vi "lock-in input sweep_1022D.vi"() -> ()   [LabVIEW 2022 SP3]
uses:
  <vilib>/Analysis/baseanly.llb/Mean (DBL).vi
  <vilib>/Utility/file.llb/Write Delimited Spreadsheet (DBL).vi
  <vilib>/Analysis/NI_AALBase.lvlib
panel:
  in  "Series Resistance":string="20kOhm"
  in  "Temperature \n& Field Function":bool=TRUE
  in  "Field Approach":i32(ring) items=["Linear", "NoOvershoot", "Oscillate"]
  in  "F Rate (Oe/s)":dbl=100.0 format="%#_13g"
  in  "Set F (Oe)":dbl format="%#_13g"
  in  "Mode":i32(ring) items=["Persistent", "Driven"]
  in  "Temperature Approach":i32(ring)=1 items=["FastSettle", "NoOvershoot"]
  in  "T  Rate (K/min)":dbl=10.0
  in  "Set  T  (K)":dbl=2.0
  in  "WaitForField":bool=TRUE
  in  "WaitForTemperature":bool=TRUE
  out "Temperature Status":i32(ring) items=["TemperatureUnknown"=0, "Stable"=1, "Tracking"=2, "Near"=5, "Chasing"=6, "Filling"=7, "Standby"=10, "Disabled"=13, "ImpedanceNotFunction"=14, "TempFailure"=15]
  out "Field Status":i32(ring) items=["MagnetUnknown"=0, "StablePersistent"=1, "WarmingSwitch"=2, "CoolingSwitch"=3, "StableDriven"=4, "Iterating"=5, "Charging"=6, "Discharging"=7, "CurrentError"=8, "MagnetFailure"=15]
  out "Field":dbl
  in  "Delay":dbl=5.0
  out "Temperature":dbl
  in  "Remote":bool=TRUE
  in  "IP Address":string="169.254.170.239"
  out "Measuring":bool
  in  "A Low Pass Filter Slope":u8(ring)=2 items=["6 dB/oct", "12 dB/oct", "18 db/oct", "24 dB/oct"]
  in  "B Low Pass Filter Slope":u8(ring)=2 items=["6 dB/oct", "12 dB/oct", "18 db/oct", "24 dB/oct"]
  in  "B Reference Source":u8(ring) items=["External", "Internal", "Internal Sweep", "Channel-A"]
  in  "B Time Constant":u8(ring)=9 items=["10 us", "30 us", "100 us", "300 us", "1 ms", "3 ms", "10 ms", "30 ms", "100 ms", "300 ms", "1 s", "3 s", "10 s", "30 s", "100 s", "300 s", "1 ks", "3 ks"]
  in  "Enable Sync Filter B (open when f<200Hz)":bool
  in  "B Sensitivity":u16(ring)=17 items=["1 nV/fA", "2 nV/fA", "5 nV/fA", "10 nV/fA", "20 nV/fA", "50 nV/fA", "100 nV/fA", "200 nV/fA", "500 nV/fA", "1 uV/pA", "2 uV/pA", "5 uV/pA", "10 uV/pA", "20 uV/pA", "50 uV/pA", "100 uV/pA", "200 uV/pA", "500 uV/pA", "1 mV/nA", "2 mV/nA", "5 mV/nA", "10 mV/nA", "20 mV/nA", "50 mV/nA", "100 mV/nA", "200 mV/nA", "500 mV/nA", "1 V/uA"]
  in  "A Sensitivity":u16(ring)=23 items=["1 nV/fA", "2 nV/fA", "5 nV/fA", "10 nV/fA", "20 nV/fA", "50 nV/fA", "100 nV/fA", "200 nV/fA", "500 nV/fA", "1 uV/pA", "2 uV/pA", "5 uV/pA", "10 uV/pA", "20 uV/pA", "50 uV/pA", "100 uV/pA", "200 uV/pA", "500 uV/pA", "1 mV/nA", "2 mV/nA", "5 mV/nA", "10 mV/nA", "20 mV/nA", "50 mV/nA", "100 mV/nA", "200 mV/nA", "500 mV/nA", "1 V/uA"]
  in  "Enable Sync Filter A (open when f<200Hz)":bool
  in  "A Time Constant":u8(ring)=9 items=["10 us", "30 us", "100 us", "300 us", "1 ms", "3 ms", "10 ms", "30 ms", "100 ms", "300 ms", "1 s", "3 s", "10 s", "30 s", "100 s", "300 s", "1 ks", "3 ks"]
  out "XY Graph 4":cluster{dbl[], dbl[]}(graph)
  in  "Phase B":u16(ring)=9 items=["X", "Y", "R", "Theta", "Frequency", "Noise", "Xh1", "Yh1", "Rh1", "Theta h1", "Xh2", "Yh2", "Rh2", "Theta h2"]
  in  "Parameter B":u16(ring)=8 items=["X", "Y", "R", "Theta", "Frequency", "Noise", "Xh1", "Yh1", "Rh1", "Theta h1", "Xh2", "Yh2", "Rh2", "Theta h2"]
  out "phase B":dbl
  in  "Clear Plot B":bool
  out "XY Graph 3":cluster{dbl[], dbl[]}(graph)
  out "para2 Measurement":dbl=1.49013e-07
  out "XY Graph 2":cluster{dbl[], dbl[]}(graph)
  in  "B Sample time (s)":dbl=0.001 min=0.001 max=100.0 step=0.001
  in  "A Sample time (s)":dbl=0.001 min=0.001 max=100.0 step=0.001
  in  "Phase A":u16(ring)=3 items=["X", "Y", "R", "Theta", "Frequency", "Noise", "Xh1", "Yh1", "Rh1", "Theta h1", "Xh2", "Yh2", "Rh2", "Theta h2"]
  in  "Parameter A":u16(ring)=2 items=["X", "Y", "R", "Theta", "Frequency", "Noise", "Xh1", "Yh1", "Rh1", "Theta h1", "Xh2", "Yh2", "Rh2", "Theta h2"]
  in  "stabilization(S)":dbl=1.0 format="%#_13g"
  in  "B frequency":dbl=267.77 format="%#_13g"
  in  "B Input Connection (0: Single-Ended)":u16(ring)=1 items=["Single-Ended Voltage", "Differential Voltage", "1 MOhm Current Gain", "100 MOhm Current Gain"]
  in  "B harmonic 1":u8=2
  in  "B harmonic 2":u8=3
  in  "B reference Manual Phase  2":dbl=-59.75
  in  "auto phase B":bool=TRUE
  in  "A frequency":dbl=267.77 format="%#_13g"
  in  "A Input Connection (0: Single-Ended)":u16(ring)=1 items=["Single-Ended Voltage", "Differential Voltage", "1 MOhm Current Gain", "100 MOhm Current Gain"]
  in  "A harmonic 1":u8=2
  in  "A harmonic 2":u8=3
  in  "A reference Manual Phase":dbl=-59.75
  in  "auto phase A":bool=TRUE
  in  "A Reference Source":u8(ring)=1 items=["External", "Internal", "Internal Sweep"]
  out "phase A":dbl
  out "loop run":i32
  in  "loop #":i32=1
  in  "Save data or not":bool=TRUE
  in  "path (folder + filename)":string="G:\\My Drive\\Opticool\\Measurement\\NLH\\f dependence\\TaI21_A1615_B166_267Hz"
  in  "Clear Plot A":bool
  out "XY Graph":cluster{dbl[], dbl[]}(graph)
  out "para1 Measurement":dbl=1.49013e-07
  out "Sine voltage":dbl format="%#_13g"
  in  "GATE STEP(mv)":i32=20
  in  "Sine Low Value (default 0V)":dbl=0.1
  in  "Sine High Value (0.001-5V)":dbl=3.5
  in  "lockin waiting (s)":dbl=0.1 format="%#_13g"
  in  "LOCKIN address":refnum<visa-resource-name>="COM3"
  # "Lock-in Setting"
  # "Channel B"
  # "Channel A"
  # "Mesurement"
  # "Sine Sweep Setting (Channel A)"
  # "Temprature and Field Setting"
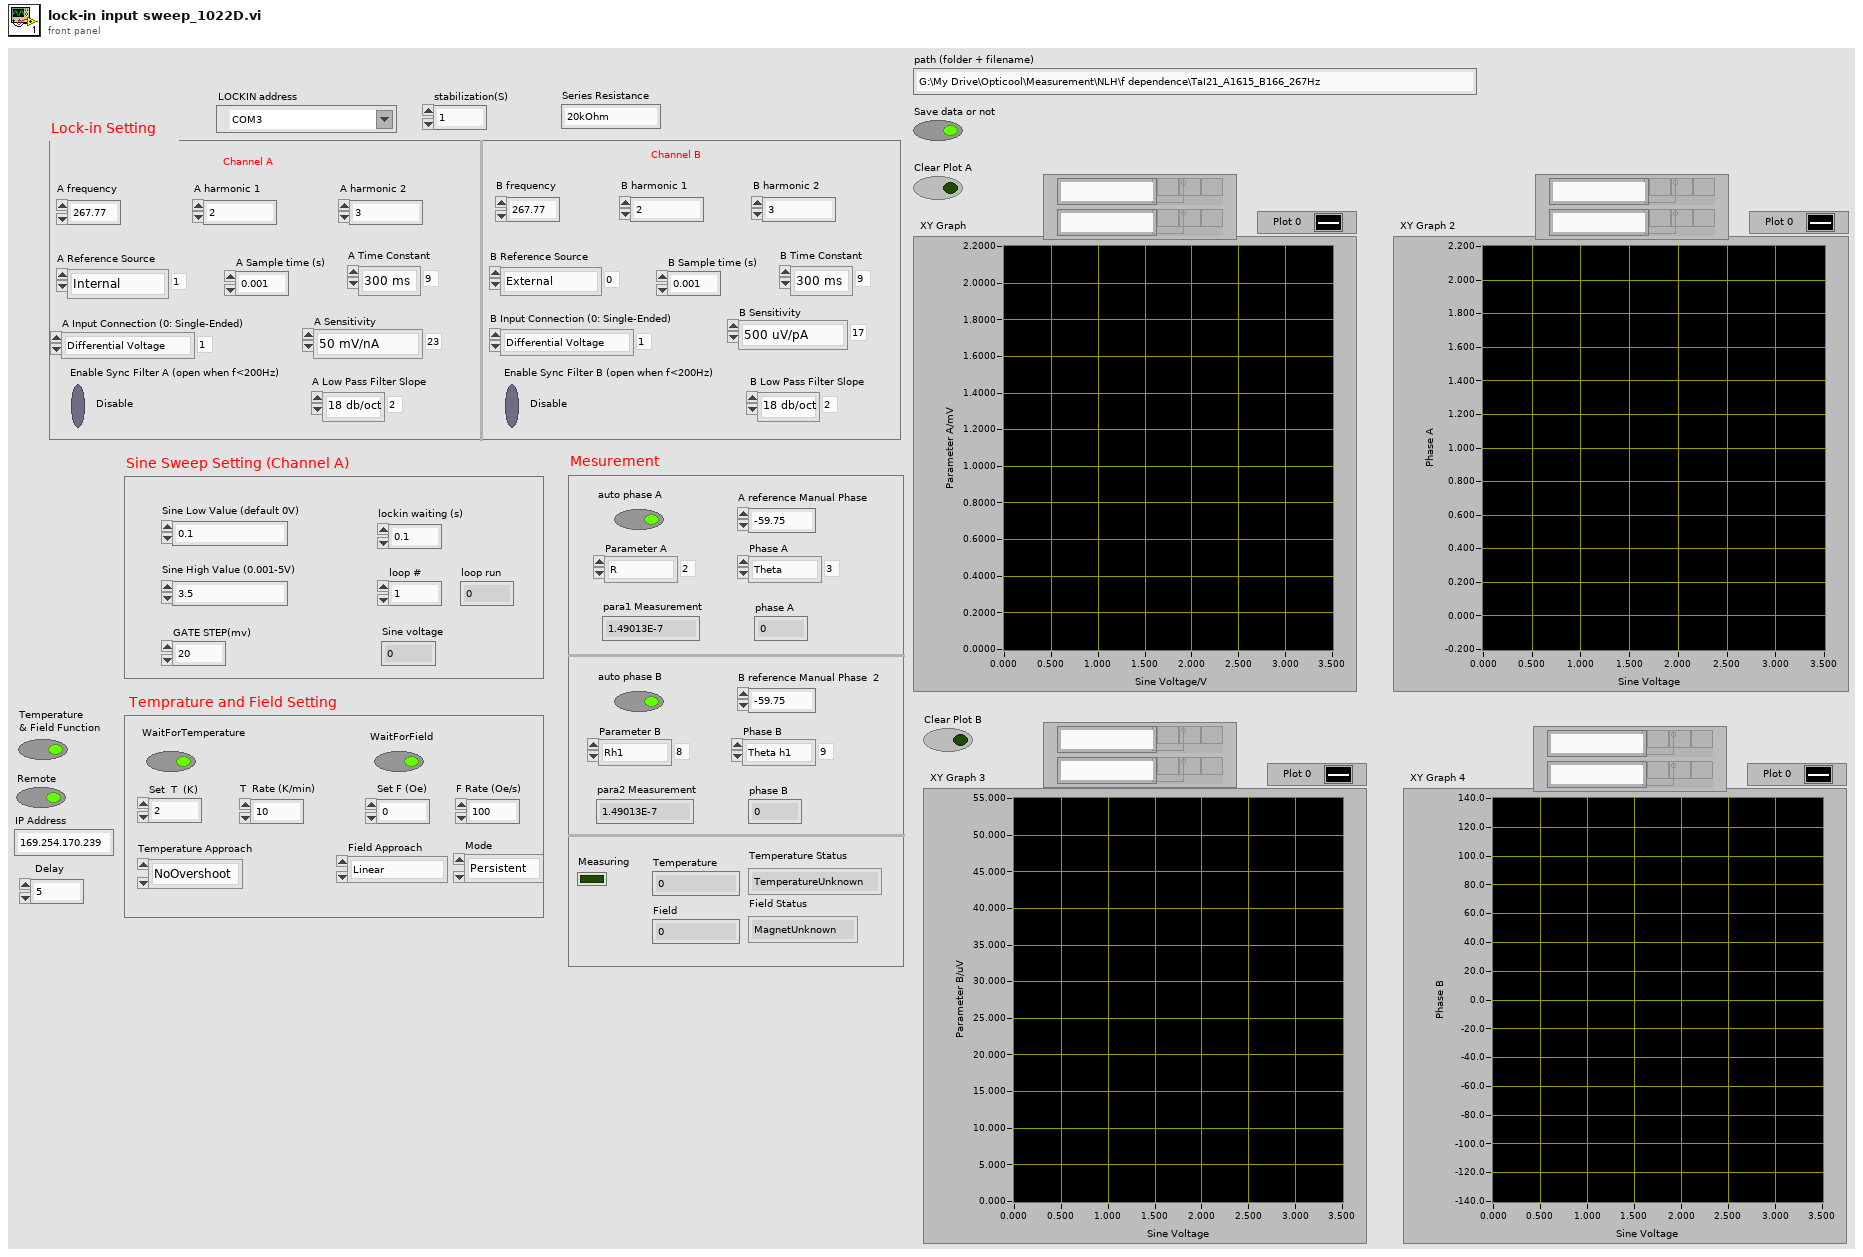
[diagram p1: front panel]
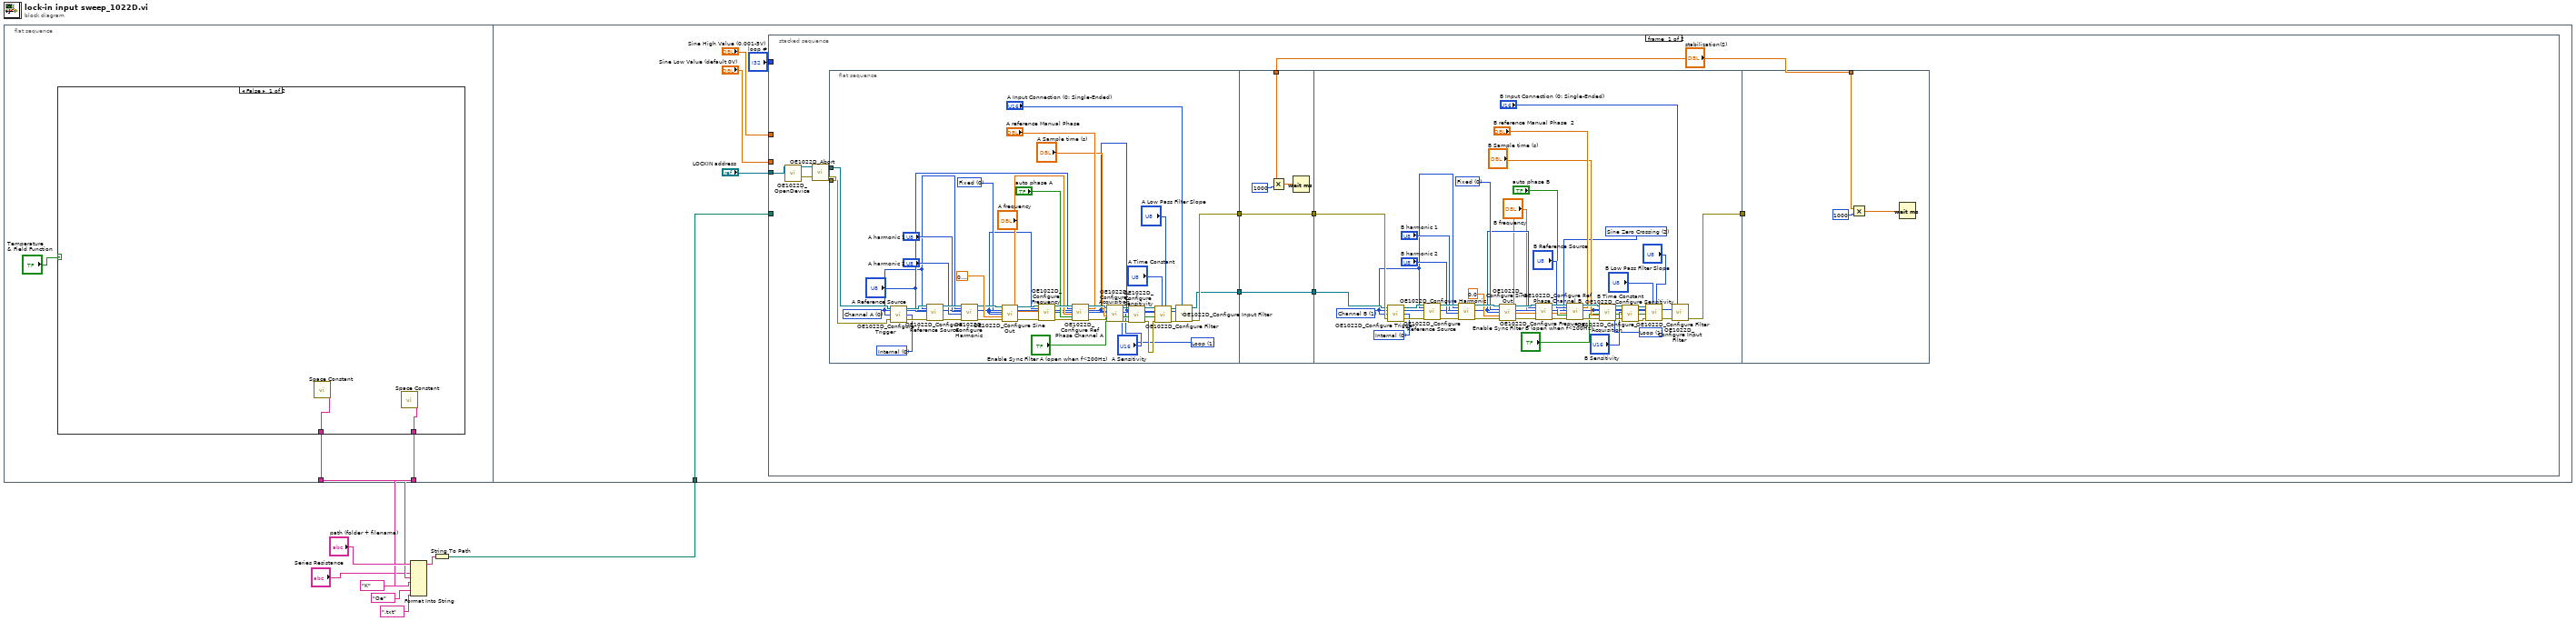
[diagram p0: block diagram]
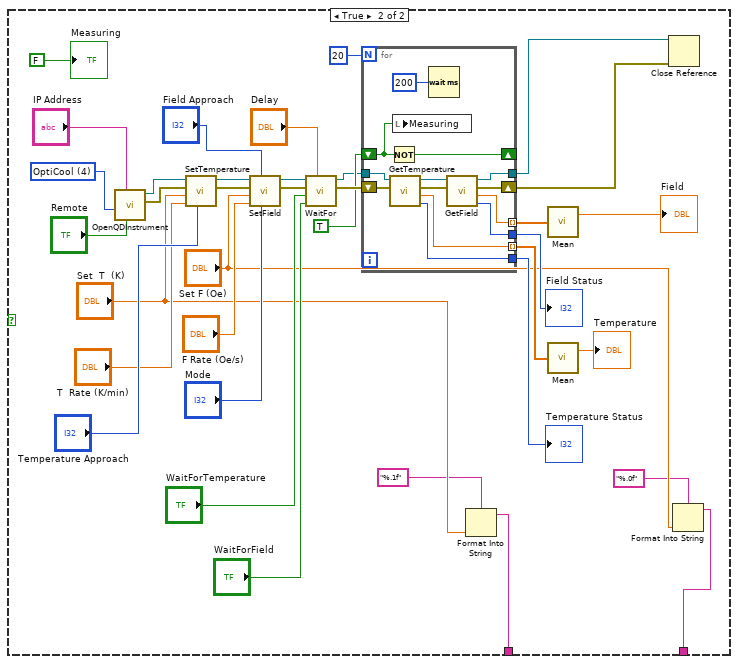
[diagram p2: hidden frame]
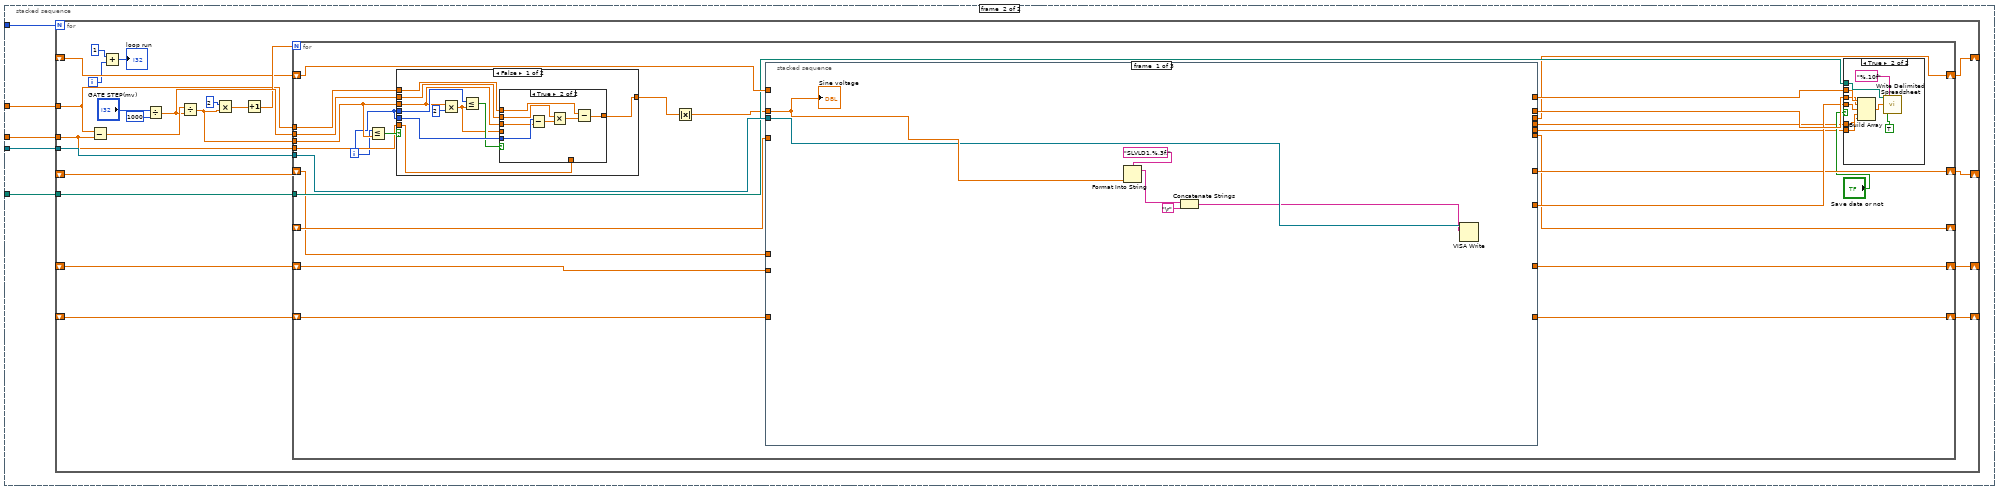
[diagram p3: hidden frame]
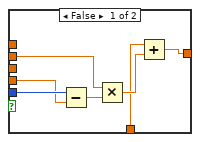
[diagram p5: hidden frame]
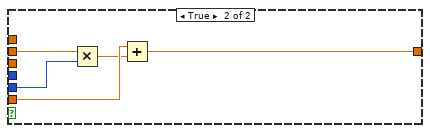
[diagram p6: hidden frame]
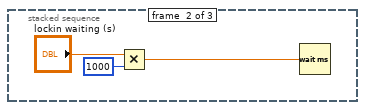
[diagram p7: hidden frame]
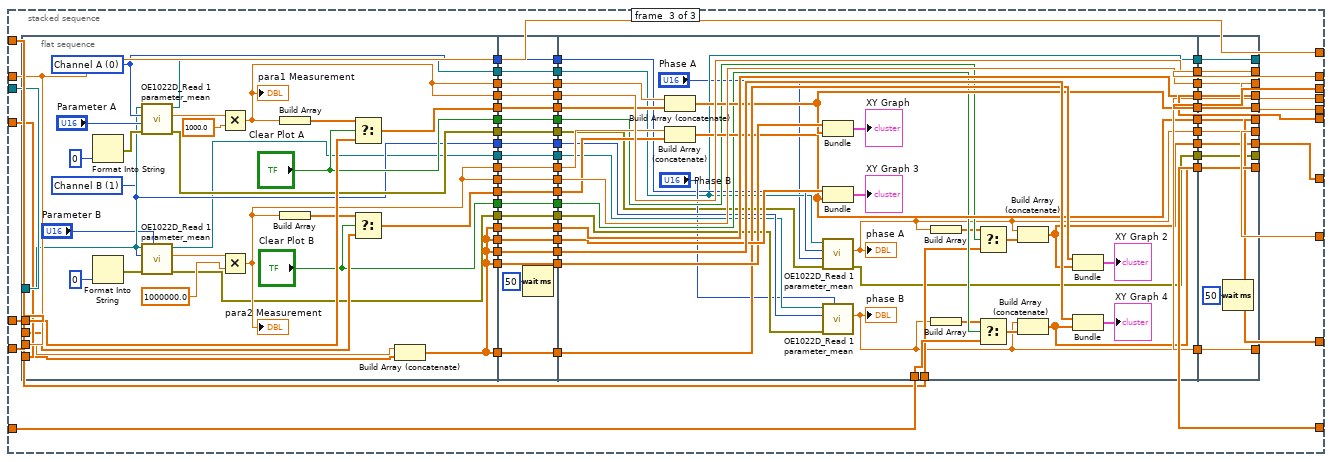
[diagram p8: hidden frame]
diagram:
  n1 = flat-sequence {
    tunnel: [w12] -> w2
    tunnel: [w11] -> w6
    tunnel: w9 -> [w65]
    frame #0 {
      n2 = case shown="False" "Temperature \n& Field Function" {
        tunnel: [w14 w16] -> w12
        tunnel: [w13 w15] -> w11
        frame False {
          n3 = call <vilib>:"Space Constant.vi"() -> ("String"=w14:string)
          n4 = call <vilib>:"Space Constant.vi"() -> ("String"=w13:string)
        }
        frame True {
          w41 = 4 items=["PPMS", "VersaLab", "DynaCool", "SVSM", "OptiCool"] ("InstrumentType")
          n5 = call "OpenQDInstrument.vi"("Remote"="Remote", "IP Address"="IP Address", "InstrumentType"=w41) -> ("error out"=w28:errorcluster, "Instrument Ref"=w29:refnum<k24>)  [unwired: 5 in]
          n6 = call "SetTemperature.vi"("Approach"="Temperature Approach", "Rate"="T  Rate (K/min)", "Temperature"="Set  T  (K)", "error in (no error)"=w28, "Instrument Ref In"=w29) -> ("error out"=w47:errorcluster, "Instrument Ref Out"=w46:refnum<k24>)  [unwired: 2 in, 1 out]
          n7 = call "SetField.vi"("Mode"="Mode", "Approach"="Field Approach", "Rate"="F Rate (Oe/s)", "Field"="Set F (Oe)", "error in (no error)"=w47, "Instrument Ref In"=w46) -> ("error out"=w24:errorcluster, "Instrument Ref Out"=w25:refnum<k24>)  [unwired: 1 in, 1 out]
          n8 = call "WaitFor.vi"("Delay"="Delay", "Wait For Field"="WaitForField", "Wait For Temperature"="WaitForTemperature", "error in (no error)"=w24, "Instrument Ref In"=w25) -> ("error out"=w40:errorcluster, "Instrument Ref Out"=w36:refnum<k24>)  [unwired: 5 in]
          n9 = for {
            N: 20 -> [_]
            shift-right: [w63] -> _
            shift-left: TRUE -> [w61]
            shift-right: [w58] -> w26
            shift-left: w40 -> [w60]
            tunnel: w36 -> [w57]
            tunnel: [w55] -> w27
            tunnel: [w52] -> w35
            tunnel: [w51] -> w34
            tunnel: [w53] -> w32 mode=indexing
            tunnel: [w54] -> w33 mode=indexing
            n10 = Not(x=w61) -> (.not. x?=w63:bool)
            n11 = call "GetTemperature.vi"("error in (no error)"=w60, "Instrument Ref In"=w57) -> ("Temperature\nStatus"=w51:i32, "Temperature"=w54:dbl, "error out"=w59:errorcluster, "Instrument Ref Out"=w56:refnum<k24>)  [unwired: 3 in, 1 out]
            n12 = local write "Measuring"(w61) -> ()
            n13 = Wait (ms)(milliseconds to wait=u32 200) -> ()  [unwired: 1 out]
            n14 = call "GetField.vi"("error in (no error)"=w59, "Instrument Ref In"=w56) -> ("Field\nStatus"=w52:i32, "Field"=w53:dbl, "error out"=w58:errorcluster, "Instrument Ref Out"=w55:refnum<k24>)  [unwired: 3 in, 1 out]
          }
          "Field Status" <- w35
          "Temperature Status" <- w34
          n15 = Format Into String(format string="%.1f", "Set  T  (K)") -> (resulting string=w16:string)  [unwired: 2 in, 1 out]
          n16 = call-poly <vilib>:"Mean.vi"("X"=w32) -> ("mean"=→"Field":dbl)  [unwired: 1 out]
          n17 = call-poly <vilib>:"Mean.vi"("X"=w33) -> ("mean"=→"Temperature":dbl)  [unwired: 1 out]
          n18 = Close Reference(reference=w27, error in (no error)=w26) -> ()  [unwired: 1 out]
          n19 = Format Into String(format string="%.0f", "Set F (Oe)") -> (resulting string=w15:string)  [unwired: 2 in, 1 out]
          "Measuring" <- FALSE
        }
      }
    }
    frame #1 {
      n20 = stacked-sequence {
        tunnel: "LOCKIN address" -> [w71 w169]
        tunnel: "Sine High Value (0.001-5V)" -> [_ w167]
        tunnel: "Sine Low Value (default 0V)" -> [_ w168]
        tunnel: w65 -> [_ w166]
        tunnel: "loop #" -> [_ w165]
        frame #0 {
          n21 = call <instrlib>:"OE1022D_OpenDevice.vi"("VISA resource name"=w71) -> ("VISA资源名称输出"=w70:refnum<visa-resource-name>, "错误输出"=w72:errorcluster)  [unwired: 17 in]
          n22 = call <instrlib>:"OE1022D_Abort.vi"("error in (no error)"=w72, "VISA resource name"=w70) -> ("error out"=w77:errorcluster, "VISA resource name out"=w78:refnum<visa-resource-name>)
          n23 = flat-sequence {
            tunnel: w78 -> [w118]
            tunnel: [w106] -> w76
            tunnel: w77 -> [w117]
            tunnel: [w94] -> w74
            tunnel: w76 -> [w123]
            tunnel: [w123] -> w75
            tunnel: w74 -> [w122]
            tunnel: [w122] -> w73
            tunnel: "stabilization(S)" -> [w119]
            tunnel: w75 -> [w144]
            tunnel: [w143] -> w79
            tunnel: w73 -> [w142]
            tunnel: w79 -> [_]
            tunnel: "stabilization(S)" -> [w162]
            frame #0 {
              w80 = u8 1 items=["Single", "Loop"] ("Sample Mode (Single/Loop)")
              w93 = u8 0 items=["Fixed", "Linear", "Log"] ("SineOut Mode")
              w95 = u16 0 items=["Internal", "External"] ("Trigger Source (0: Internal)")
              w84 = u8 0 items=["Channel A", "Channel B"] ("OE1022D A/B")
              n24 = call <instrlib>:"OE1022D_Configure Trigger.vi"("Trigger Source (0: Internal)"=w95, "error in (no error)   2"=w117, "OE1022D A/B"=w84, "VISA resource name   2"=w118) -> ("error out   2"=w111:errorcluster, "VISA resource name out   2"=w112:refnum<visa-resource-name>)
              n25 = call <instrlib>:"OE1022D_Configure Reference Source.vi"("VISA resource name"=w112, "OE1022D A/B"=w84, "Reference Source"="A Reference Source", "error in (no error)"=w111) -> ("VISA resource name out"=w110:refnum<visa-resource-name>, "error out"=w108:errorcluster)  [unwired: 14 in]
              n26 = call <instrlib>:"OE1022D_Configure Harmonic.vi"("VISA resource name"=w110, "OE1022D A/B"=w84, "Harmonic 1"="A harmonic 1", "Harmonic 2"="A harmonic 2", "error in (no error)"=w108) -> ("VISA resource name out"=w109:refnum<visa-resource-name>, "error out"=w107:errorcluster)  [unwired: 13 in]
              n27 = call <instrlib>:"OE1022D_Configure Sine Out.vi"("VISA resource name"=w109, "SineOut Mode"=w93, "OE1022D A/B"=w84, "Sine Output Amplitude (V)"=sgl 0.1, "error in (no error)"=w107) -> ("VISA resource name out"=w115:refnum<visa-resource-name>, "error out"=w114:errorcluster)  [unwired: 9 in]
              n28 = call <instrlib>:"OE1022D_Configure Frequency.vi"("VISA resource name"=w115, "OE1022D A/B"=w84, "Internal Frequency(Hz)"="A frequency", "error in (no error)"=w114) -> ("VISA resource name out"=w105:refnum<visa-resource-name>, "error out"=w102:errorcluster)  [unwired: 14 in]
              n29 = call <instrlib>:"OE1022D_Configure Ref Phase Channel A.vi"("VISA resource name"=w105, "Reference Source"="A Reference Source", "Internal Frequency(Hz)"="A frequency", "Auto Phase (T: Enabled)"="auto phase A", "error in (no error)"=w102, "Manual Phase  (degree)"="A reference Manual Phase") -> ("VISA resource name out"=w104:refnum<visa-resource-name>, "error out"=w103:errorcluster)  [unwired: 12 in]
              n30 = call <instrlib>:"OE1022D_Configure_Acquisition.vi"("VISA resource name"=w104, "OE1022D A/B"=w84, "Sample time (s)"="A Sample time (s)", "error in (no error)"=w103, "Sample Mode (Single/Loop)"=w80) -> ("VISA resource name out"=w87:refnum<visa-resource-name>, "error out"=w86:errorcluster)  [unwired: 3 in]
              n31 = call <instrlib>:"OE1022D_Configure Sensitivity.vi"("VISA resource name"=w87, "OE1022D A/B"=w84, "Sensitivity"="A Sensitivity", "error in (no error)"=w86) -> ("VISA resource name out"=w91:refnum<visa-resource-name>, "error out"=w90:errorcluster)  [unwired: 14 in]
              n32 = call <instrlib>:"OE1022D_Configure Filter.vi"("Low Pass Filter Slope (1: 12dB/oct)"="A Low Pass Filter Slope", "Time Constant (8: 100ms)"="A Time Constant", "error in (no error)"=w90, "Enable Sync Filter (F: Disable)"="Enable Sync Filter A (open when f<200Hz)", "OE1022D A/B"=w84, "VISA resource name"=w91) -> ("error out"=w88:errorcluster, "VISA resource name out"=w89:refnum<visa-resource-name>)  [unwired: 4 in]
              n33 = call <instrlib>:"OE1022D_Configure Input Filter.vi"("VISA resource name"=w89, "Input Source"="A Input Connection (0: Single-Ended)", "OE1022D A/B"=w84, "error in (no error)"=w88) -> ("VISA resource name out"=w94:refnum<visa-resource-name>, "error out"=w106:errorcluster)  [unwired: 10 in]
            }
            frame #1 {
              n34 = Multiply(x=w119, y=1000) -> (x*y=w121:dbl)
              n35 = Wait (ms)(milliseconds to wait=w121) -> ()  [unwired: 1 out]
            }
            frame #2 {
              w124 = u8 1 items=["Single", "Loop"] ("Sample Mode (Single/Loop)")
              w126 = u8 2 items=["TTL Pos", "TTL Neg", "Sine Zero Crossing"] ("External Ref Trigger")
              w139 = u8 0 items=["Fixed", "Linear", "Log"] ("SineOut Mode")
              w145 = u16 0 items=["Internal", "External"] ("Trigger Source (0: Internal)")
              w131 = u8 1 items=["Channel A", "Channel B"] ("OE1022D A/B")
              n36 = call <instrlib>:"OE1022D_Configure Trigger.vi"("Trigger Source (0: Internal)"=w145, "error in (no error)   2"=w144, "OE1022D A/B"=w131, "VISA resource name   2"=w142) -> ("error out   2"=w157:errorcluster, "VISA resource name out   2"=w158:refnum<visa-resource-name>)
              n37 = call <instrlib>:"OE1022D_Configure Reference Source.vi"("VISA resource name"=w158, "OE1022D A/B"=w131, "error in (no error)"=w157) -> ("VISA resource name out"=w156:refnum<visa-resource-name>, "error out"=w154:errorcluster)  [unwired: 15 in]
              n38 = call <instrlib>:"OE1022D_Configure Harmonic.vi"("VISA resource name"=w156, "OE1022D A/B"=w131, "Harmonic 1"="B harmonic 1", "Harmonic 2"="B harmonic 2", "error in (no error)"=w154) -> ("VISA resource name out"=w155:refnum<visa-resource-name>, "error out"=w153:errorcluster)  [unwired: 13 in]
              n39 = call <instrlib>:"OE1022D_Configure Sine Out.vi"("VISA resource name"=w155, "SineOut Mode"=w139, "OE1022D A/B"=w131, "Sine Output Amplitude (V)"=sgl 0.0, "error in (no error)"=w153) -> ("VISA resource name out"=w160:refnum<visa-resource-name>, "error out"=w159:errorcluster)  [unwired: 9 in]
              n40 = call <instrlib>:"OE1022D_Configure Frequency.vi"("VISA resource name"=w160, "OE1022D A/B"=w131, "Internal Frequency(Hz)"="B frequency", "error in (no error)"=w159) -> ("VISA resource name out"=w152:refnum<visa-resource-name>, "error out"=w149:errorcluster)  [unwired: 14 in]
              n41 = call <instrlib>:"OE1022D_Configure Ref Phase Channel B.vi"("VISA resource name"=w152, "Reference Source"="B Reference Source", "External Ref Trigger"=w126, "Internal Frequency(Hz)"="B frequency", "Auto Phase (T: Enabled)"="auto phase B", "error in (no error)"=w149, "Manual Phase  (degree)"="B reference Manual Phase  2") -> ("VISA resource name out"=w151:refnum<visa-resource-name>, "error out"=w150:errorcluster)  [unwired: 11 in]
              n42 = call <instrlib>:"OE1022D_Configure_Acquisition.vi"("VISA resource name"=w151, "OE1022D A/B"=w131, "Sample time (s)"="B Sample time (s)", "error in (no error)"=w150, "Sample Mode (Single/Loop)"=w124) -> ("VISA resource name out"=w132:refnum<visa-resource-name>, "error out"=w133:errorcluster)  [unwired: 3 in]
              n43 = call <instrlib>:"OE1022D_Configure Sensitivity.vi"("VISA resource name"=w132, "OE1022D A/B"=w131, "Sensitivity"="B Sensitivity", "error in (no error)"=w133) -> ("VISA resource name out"=w136:refnum<visa-resource-name>, "error out"=w135:errorcluster)  [unwired: 14 in]
              n44 = call <instrlib>:"OE1022D_Configure Filter.vi"("Low Pass Filter Slope (1: 12dB/oct)"="B Low Pass Filter Slope", "Time Constant (8: 100ms)"="B Time Constant", "error in (no error)"=w135, "Enable Sync Filter (F: Disable)"="Enable Sync Filter B (open when f<200Hz)", "OE1022D A/B"=w131, "VISA resource name"=w136) -> ("error out"=w134:errorcluster)  [unwired: 4 in, 1 out]
              n45 = call <instrlib>:"OE1022D_Configure Input Filter.vi"("Input Source"="B Input Connection (0: Single-Ended)", "OE1022D A/B"=w131, "error in (no error)"=w134) -> ("error out"=w143:errorcluster)  [unwired: 11 in, 1 out]
            }
            frame #3 {
              n46 = Multiply(x=w162, y=1000) -> (x*y=w164:dbl)
              n47 = Wait (ms)(milliseconds to wait=w164) -> ()  [unwired: 1 out]
            }
          }
        }
        frame #1 {
          n48 = for {
            N: w165 -> [_]
            tunnel: w169 -> [w192]
            tunnel: w168 -> [w186]
            tunnel: w167 -> [w176]
            tunnel: w166 -> [w185]
            shift-right: [w181] -> _
            shift-left: _ -> [w180]
            shift-right: [w175] -> _
            shift-left: _ -> [w174]
            shift-right: [w173] -> _
            shift-left: _ -> [w172]
            shift-right: [w171] -> _
            shift-left: _ -> [w170]
            i -> [w178]
            n49 = Subtract(x=w176, y=w186) -> (x-y=w188:dbl)
            n50 = Add(x=1, y=w178) -> (x+y=→"loop run":i32)
            n51 = Divide(x="GATE STEP(mv)", y=1000) -> (x/y=w187:dbl)
            n52 = Divide(x=w188, y=w187) -> (x/y=w184:dbl)
            n53 = Multiply(x=2, y=w184) -> (x*y=w183:dbl)
            n54 = Increment(x=w183) -> (x+1=w182:dbl)
            n55 = for {
              N: w182 -> [_]
              tunnel: w192 -> [w218]
              tunnel: w187 -> [w214]
              shift-right: [w200] -> w181
              shift-left: w180 -> [w217]
              tunnel: w184 -> [w212]
              tunnel: w186 -> [w215]
              tunnel: w176 -> [w213]
              tunnel: w185 -> [w208]
              shift-right: [w199] -> _
              shift-left: _ -> [w204]
              shift-right: [w203] -> w175
              shift-left: w174 -> [w202]
              shift-right: [w198] -> w173
              shift-left: w172 -> [w197]
              shift-right: [w196] -> w171
              shift-left: w170 -> [w195]
              i -> [w211]
              n56 = Less Or Equal?(x=w211, y=w212) -> (x <= y?=w216:bool)
              n57 = case shown="False" w216 {
                tunnel: w215 -> [w228 w256]
                tunnel: w211 -> [w237 w255]
                tunnel: w214 -> [w236 w254]
                tunnel: [w234 w252] -> w207
                tunnel: w213 -> [w235 _]
                tunnel: w212 -> [w230 _]
                tunnel: w211 -> [w233 _]
                frame False {
                  n58 = Multiply(x=w230, y=2) -> (x*y=w229:dbl)
                  n59 = Less Or Equal?(x=w233, y=w229) -> (x <= y?=w231:bool)
                  n60 = case shown="True" w231 {
                    tunnel: w237 -> [w244 w251]
                    tunnel: w236 -> [w242 w249]
                    tunnel: w235 -> [_ w247]
                    tunnel: [w240 w246] -> w234
                    tunnel: w230 -> [_ w245]
                    tunnel: w229 -> [w239 _]
                    tunnel: w228 -> [w238 _]
                    frame False {
                      n61 = Subtract(x=w244, y=w239) -> (x-y=w243:dbl)
                      n62 = Multiply(x=w242, y=w243) -> (x*y=w241:dbl)
                      n63 = Add(x=w238, y=w241) -> (x+y=w240:dbl)
                    }
                    frame True {
                      n64 = Subtract(x=w251, y=w245) -> (x-y=w250:dbl)
                      n65 = Multiply(x=w249, y=w250) -> (x*y=w248:dbl)
                      n66 = Subtract(x=w247, y=w248) -> (x-y=w246:dbl)
                    }
                  }
                }
                frame True {
                  n67 = Multiply(x=w254, y=w255) -> (x*y=w253:dbl)
                  n68 = Add(x=w256, y=w253) -> (x+y=w252:dbl)
                }
              }
              n69 = Absolute Value(x=w207) -> (abs(x)=w206:dbl)
              n70 = stacked-sequence {
                tunnel: w218 -> [w260 _ w328]
                tunnel: w206 -> [w261 _ w326]
                tunnel: w217 -> [_ _ w330]
                tunnel: [_ _ w329] -> w200
                tunnel: [_ _ w327] -> w210
                tunnel: [_ _ w326] -> w209
                tunnel: [_ _ w325] -> w199
                tunnel: w204 -> [_ _ w324]
                tunnel: [_ _ w323] -> w205
                tunnel: [_ _ w322] -> w203
                tunnel: w202 -> [_ _ w315]
                tunnel: [_ _ w321] -> w198
                tunnel: w197 -> [_ _ w316]
                tunnel: [_ _ w320] -> w196
                tunnel: w195 -> [_ _ w319]
                tunnel: [_ _ w318] -> w194
                tunnel: [_ _ w317] -> w193
                frame #0 {
                  n71 = Format Into String(format string="SLVLD1,%.3f;", w261) -> (resulting string=w258:string)  [unwired: 2 in, 1 out]
                  n72 = Concatenate Strings(w258, "\r") -> (w257:string)
                  n73 = VISA Write(VISA resource name=w260, write buffer=w257) -> ()  [unwired: 1 in, 3 out]
                  "Sine voltage" <- w261
                }
                frame #1 {
                  n74 = Multiply(x="lockin waiting (s)", y=1000) -> (x*y=w265:dbl)
                  n75 = Wait (ms)(milliseconds to wait=w265) -> ()  [unwired: 1 out]
                }
                frame #2 {
                  n76 = flat-sequence {
                    tunnel: w330 -> [w358]
                    tunnel: w328 -> [w337]
                    tunnel: w326 -> [w357]
                    tunnel: w324 -> [w356]
                    tunnel: w319 -> [w350]
                    tunnel: [w354] -> w314
                    tunnel: [w346] -> w312
                    tunnel: [w347] -> w310
                    tunnel: [w344] -> w308
                    tunnel: [w347] -> w306
                    tunnel: [w347] -> w304
                    tunnel: [w347] -> w302
                    tunnel: [w347] -> w300
                    tunnel: [w346] -> w298
                    tunnel: [w345] -> w296
                    tunnel: [w344] -> w294
                    tunnel: [w343] -> w292
                    tunnel: ["Clear Plot B"] -> w290
                    tunnel: ["Clear Plot A"] -> w288
                    tunnel: [w333] -> w286
                    tunnel: [w335] -> w284
                    tunnel: [w334] -> w282
                    tunnel: [w340] -> w280
                    tunnel: [w339] -> w278
                    tunnel: w314 -> [w380]
                    tunnel: [w380] -> w313
                    tunnel: w312 -> [w379]
                    tunnel: [w379] -> w311
                    tunnel: w310 -> [w378]
                    tunnel: [w378] -> w309
                    tunnel: w308 -> [w377]
                    tunnel: [w377] -> w307
                    tunnel: w306 -> [w376]
                    tunnel: [w376] -> w305
                    tunnel: w304 -> [w375]
                    tunnel: [w375] -> w303
                    tunnel: w302 -> [w374]
                    tunnel: [w374] -> w301
                    tunnel: w300 -> [w373]
                    tunnel: [w373] -> w299
                    tunnel: w298 -> [w372]
                    tunnel: [w372] -> w297
                    tunnel: w296 -> [w371]
                    tunnel: [w371] -> w295
                    tunnel: w294 -> [w370]
                    tunnel: [w370] -> w293
                    tunnel: w292 -> [w369]
                    tunnel: [w369] -> w291
                    tunnel: w290 -> [w368]
                    tunnel: [w368] -> w289
                    tunnel: w288 -> [w367]
                    tunnel: [w367] -> w287
                    tunnel: w286 -> [w366]
                    tunnel: [w366] -> w285
                    tunnel: w284 -> [w365]
                    tunnel: [w365] -> w283
                    tunnel: w282 -> [w364]
                    tunnel: [w364] -> w281
                    tunnel: w280 -> [w363]
                    tunnel: [w363] -> w279
                    tunnel: w278 -> [w362]
                    tunnel: [w362] -> w277
                    tunnel: w313 -> [w384]
                    tunnel: w311 -> [w418]
                    tunnel: w309 -> [w417]
                    tunnel: w307 -> [w416]
                    tunnel: w305 -> [w415]
                    tunnel: w303 -> [w413]
                    tunnel: w301 -> [w411]
                    tunnel: w299 -> [w409]
                    tunnel: w297 -> [w406]
                    tunnel: w295 -> [w405]
                    tunnel: w293 -> [w402]
                    tunnel: w291 -> [w401]
                    tunnel: w316 -> [w399]
                    tunnel: w289 -> [w398]
                    tunnel: w315 -> [w396]
                    tunnel: w287 -> [w395]
                    tunnel: w285 -> [w391]
                    tunnel: w283 -> [w390]
                    tunnel: w281 -> [w389]
                    tunnel: w279 -> [w386]
                    tunnel: w277 -> [w385]
                    tunnel: [w384] -> w276
                    tunnel: [w404] -> w275
                    tunnel: [w418] -> w274
                    tunnel: [w417] -> w273
                    tunnel: [w382] -> w272
                    tunnel: [w383] -> w271
                    tunnel: [w407] -> w270
                    tunnel: [w403] -> w269
                    tunnel: [w400] -> w268
                    tunnel: [w416] -> w267
                    tunnel: [w388] -> w266
                    tunnel: [w420] -> w317
                    tunnel: [w421] -> w318
                    tunnel: [w422] -> w320
                    tunnel: [w423] -> w321
                    tunnel: [w424] -> w322
                    tunnel: [w425] -> _
                    tunnel: [w426] -> w323
                    tunnel: [w427] -> w325
                    tunnel: [w428] -> w327
                    tunnel: [w429] -> w329
                    tunnel: [w430] -> _
                    tunnel: w276 -> [w430]
                    tunnel: w275 -> [w429]
                    tunnel: w274 -> [w428]
                    tunnel: w273 -> [w427]
                    tunnel: w272 -> [w426]
                    tunnel: w271 -> [w425]
                    tunnel: w270 -> [w424]
                    tunnel: w269 -> [w423]
                    tunnel: w268 -> [w422]
                    tunnel: w267 -> [w421]
                    tunnel: w266 -> [w420]
                    frame #0 {
                      w335 = u8 1 items=["Channel A", "Channel B"] ("Channel A/B for Parameter1")
                      w339 = u8 0 items=["Channel A", "Channel B"] ("Channel A/B for Parameter1")
                      n77 = Format Into String(0) -> (error out=w355:errorcluster)  [unwired: 3 in, 1 out]
                      n78 = Format Into String(0) -> (error out=w336:errorcluster)  [unwired: 3 in, 1 out]
                      n79 = call <instrlib>:"OE1022D_Read 1 parameter_mean.vi"("错误输入（无错误）"=w355, "Parameter"="Parameter A", "Channel (0: A)"=w339, "VISA resource name"=w337) -> ("error out"=w340:errorcluster, "Measurement"=w348:dbl, "VISA resource name out"=w354:refnum<visa-resource-name>)  [unwired: 5 in]
                      n80 = call <instrlib>:"OE1022D_Read 1 parameter_mean.vi"("Parameter 2"="Parameter B", "错误输入（无错误）"=w336, "Channel (0: A)"=w335, "VISA resource name"=w337) -> ("error out"=w333:errorcluster, "Measurement"=w332:dbl, "VISA resource name out"=w334:refnum<visa-resource-name>)  [unwired: 5 in]
                      n81 = Multiply(x=w348, y=1000.0) -> (x*y=w346:dbl)
                      "para1 Measurement" <- w346
                      n82 = Multiply(x=w332, y=1000000.0) -> (x*y=w344:dbl)
                      "para2 Measurement" <- w344
                      n83 = Build Array(w346) -> (w359:dbl[])
                      n84 = Build Array(w344) -> (w351:dbl[])
                      n85 = Select(t=w359, s="Clear Plot A", f=w358) -> (s? t:f=w345:dbl[])
                      n86 = Select(t=w351, s="Clear Plot B", f=w350) -> (s? t:f=w343:dbl[])
                      n87 = Build Array (concatenate)(w357, w356) -> (w347:dbl[])
                    }
                    frame #1 {
                      n88 = Wait (ms)(milliseconds to wait=u32 50) -> ()  [unwired: 1 out]
                    }
                    frame #2 {
                      n89 = Build Array (concatenate)(w406, w405) -> (w404:dbl[])
                      n90 = Build Array (concatenate)(w402, w401) -> (w400:dbl[])
                      n91 = Bundle(w411, w404) -> (→"XY Graph":cluster{dbl[], dbl[]})  [unwired: 1 in]
                      n92 = Bundle(w413, w400) -> (→"XY Graph 3":cluster{dbl[], dbl[]})  [unwired: 1 in]
                      n93 = call <instrlib>:"OE1022D_Read 1 parameter_mean.vi"("错误输入（无错误）"=w386, "Parameter"="Phase A", "Channel (0: A)"=w385, "VISA resource name"=w384) -> ("error out"=w383:errorcluster, "Measurement"=w382:dbl)  [unwired: 5 in, 1 out]
                      "phase A" <- w382
                      n94 = call <instrlib>:"OE1022D_Read 1 parameter_mean.vi"("Parameter 2"="Phase B", "错误输入（无错误）"=w391, "Channel (0: A)"=w390, "VISA resource name"=w389) -> ("Measurement"=w388:dbl)  [unwired: 5 in, 2 out]
                      "phase B" <- w388
                      n95 = Build Array(w382) -> (w392:dbl[])
                      n96 = Build Array(w388) -> (w393:dbl[])
                      n97 = Select(t=w392, s=w395, f=w396) -> (s? t:f=w394:dbl[])
                      n98 = Select(t=w393, s=w398, f=w399) -> (s? t:f=w397:dbl[])
                      n99 = Build Array (concatenate)(w382, w394) -> (w407:dbl[])
                      n100 = Build Array (concatenate)(w388, w397) -> (w403:dbl[])
                      n101 = Bundle(w409, w407) -> (→"XY Graph 2":cluster{dbl[], dbl[]})  [unwired: 1 in]
                      n102 = Bundle(w415, w403) -> (→"XY Graph 4":cluster{dbl[], dbl[]})  [unwired: 1 in]
                    }
                    frame #3 {
                      n103 = Wait (ms)(milliseconds to wait=u32 50) -> ()  [unwired: 1 out]
                    }
                  }
                }
              }
              n104 = case shown="True" "Save data or not" {
                tunnel: w210 -> [_ w222]
                tunnel: w209 -> [_ w227]
                tunnel: w208 -> [_ w225]
                tunnel: w205 -> [_ w221]
                tunnel: w194 -> [_ w220]
                tunnel: w193 -> [_ w219]
                frame False {
                }
                frame True {
                  n105 = Build Array(w227, w222, w221, w220, w219) -> (w224:dbl[])
                  n106 = call-poly <vilib>:"Write Delimited Spreadsheet.vi"("file path (dialog if empty)"=w225, "format (%.3f)"="%.10f", "1D data"=w224, "append to file? (new file:F)"=TRUE) -> ()  [unwired: 10 in, 2 out]
                }
              }
            }
          }
        }
      }
    }
  }
  n107 = Format Into String(initial string="path (folder + filename)", "Series Resistance", w2, "K", w6, "Oe", ".txt") -> (resulting string=w3:string)  [unwired: 2 in, 1 out]
  n108 = String To Path(string=w3) -> (path=w9:path)
